vi "Login Dialog.vi"() -> (0 "管理员":bool, 2 "Success?":bool)   [LabVIEW 2015]
uses:
  <vilib>/Utility/miscctls.llb/LVPointTypeDef.ctl
  Global.vi
panel:
  in  "注册":bool
  in  "登录":bool
  in  "注销":bool
  in  "Password":string caption="密   码:"
  in  "UserName":string caption="用户名:"
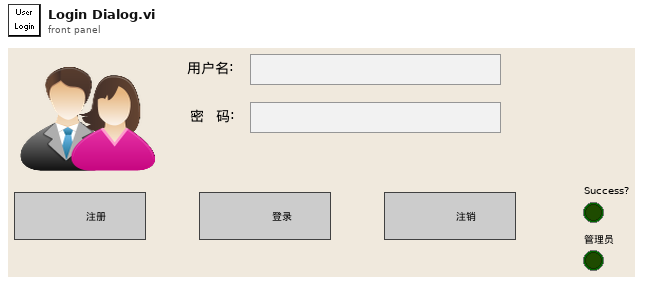
[diagram p1: front panel]
types:
  T1 = typedef "LVPointTypeDef.ctl" = cluster{"Horizontal":i16, "Vertical":i16}
  T2 = enum8{"Enabled", "Disabled", "Disabled and Grayed Out"}
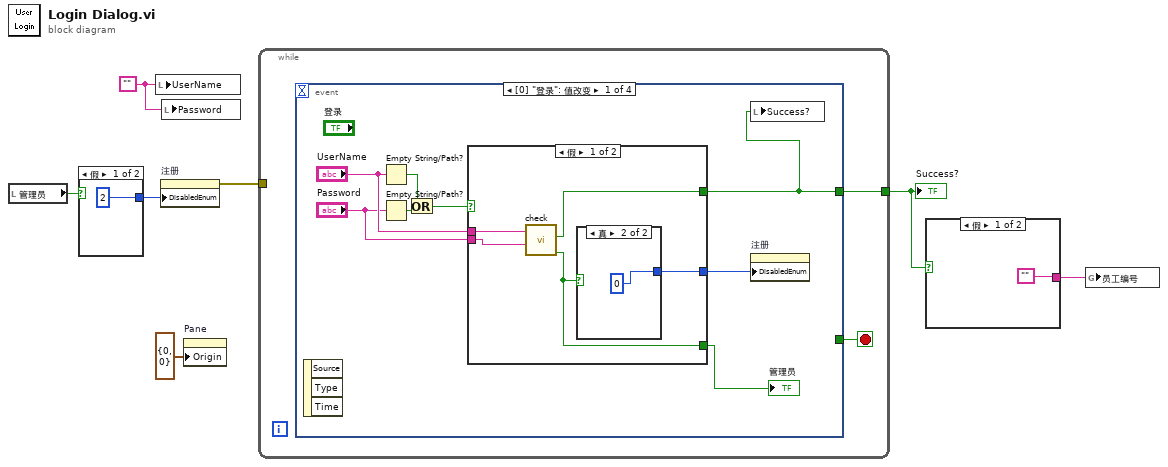
[diagram p0: block diagram]
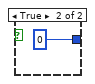
[diagram p2: hidden frame]
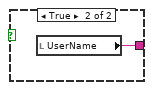
[diagram p3: hidden frame]
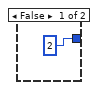
[diagram p4: hidden frame]
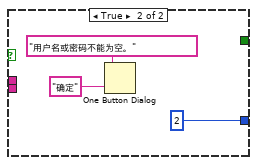
[diagram p5: hidden frame]
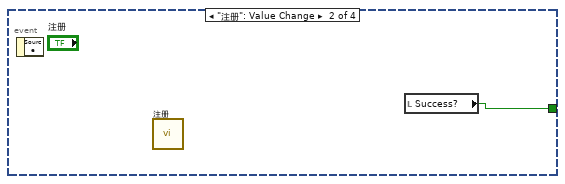
[diagram p6: hidden frame]
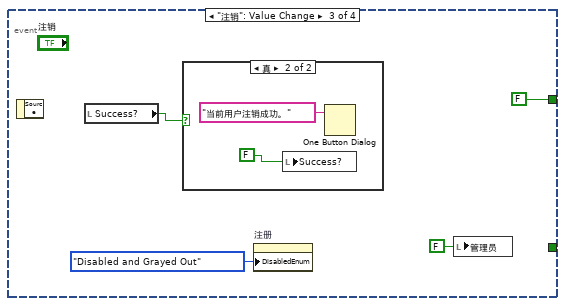
[diagram p7: hidden frame]
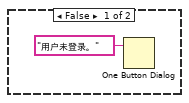
[diagram p8: hidden frame]
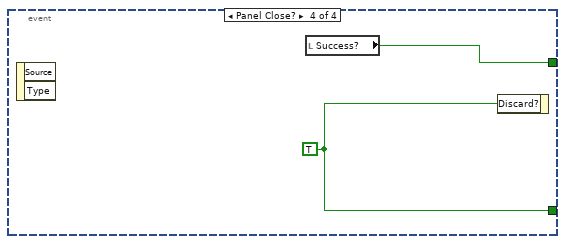
[diagram p9: hidden frame]
diagram:
  w6 = ""
  n1 = local read "管理员"() -> (w3:bool)
  n2 = case shown="假" w3 {
    tunnel: [2 0] -> w2
    frame False {
    }
    frame True {
    }
  }
  n3 = local write "UserName"(w6) -> ()
  n4 = property on="注册" class="Bool"("DisabledEnum"=w2) -> (error out=w1:errorcluster)  [unwired: 2 in, 1 out]
  n5 = local write "Password"(w6) -> ()
  n6 = property on="Pane" class="Pane"("Origin"=T1 {"Horizontal"=0, "Vertical"=0}) -> ()  [unwired: 2 in, 2 out]
  n7 = while {
    tunnel: [w10] -> w5
    tunnel: w1 -> [_]
    stop <- w11 stop-if-true
    n8 = event shown="[0] \"登录\": 值改变" {
      selector: _ -> [_ _ _ _]
      dyn-events: _ -> [_ _ _ _]
      timeout: _ -> [_ _ _ _]
      tunnel: [_ _ _ w39] -> w11
      tunnel: [w14 w30 FALSE ("Success?") w38] -> w10
      event "登录": Value Change {
        n9 = event-data() -> ()  [unwired: 1 in, 3 out]
        n10 = Empty String/Path?(string/path="UserName") -> (empty?=w18:bool)
        n11 = Empty String/Path?(string/path="Password") -> (empty?=w19:bool)
        n12 = Or(x=w18, y=w19) -> (x .or. y?=w17:bool)
        n13 = case shown="假" w17 {
          tunnel: "UserName" -> [w24 _]
          tunnel: "Password" -> [w23 _]
          tunnel: [w22 _] -> w14
          tunnel: [w21 2] -> w13
          tunnel: [w20 _] -> w12
          frame False {
            n14 = call "check.vi"("Password"=w23, "UserName"=w24) -> ("管理员"=w20:bool, "Success?"=w22:bool)  [unwired: 8 in]
            n15 = case shown="真" w20 {
              tunnel: [2 0] -> w21
              frame False {
              }
              frame True {
              }
            }
          }
          frame True {
            n16 = One Button Dialog(message="用户名或密码不能为空。", button name ("OK")="确定") -> ()  [unwired: 1 out]
          }
        }
        "管理员" <- w12
        n17 = local write "Success?"(w14) -> ()
        n18 = property on="注册" class="Bool"("DisabledEnum"=w13) -> ()  [unwired: 2 in, 2 out]
      }
      event "注册": Value Change {
        n19 = event-data() -> ()  [unwired: 1 in, 1 out]
        n20 = call "注册.vi"() -> ()  [unwired: 12 in]
        n21 = local read "Success?"() -> (w30:bool)
      }
      event "注销": Value Change {
        n22 = event-data() -> ()  [unwired: 1 in, 1 out]
        n23 = local read "Success?"() -> (w33:bool)
        n24 = case shown="真" w33 {
          frame False {
            n25 = One Button Dialog(message="用户未登录。" ("消息")) -> ()  [unwired: 1 in, 1 out]
          }
          frame True {
            n26 = local write "Success?"(FALSE ("Success?")) -> ()
            n27 = One Button Dialog(message="当前用户注销成功。" ("消息")) -> ()  [unwired: 1 in, 1 out]
          }
        }
        n28 = property on="注册" class="Bool"("DisabledEnum"=T2."Disabled and Grayed Out" ("禁用")) -> ()  [unwired: 2 in, 2 out]
        n29 = local write "管理员"(FALSE ("管理员")) -> ()
      }
      event Panel Close? {
        w39 = TRUE
        n30 = event-data() -> ()  [unwired: 1 in, 2 out]
        n31 = local read "Success?"() -> (w38:bool)
        n32 = event-data("Discard?"=w39) -> ()  [unwired: 1 in, 1 out]
      }
    }
  }
  "Success?" <- w5
  n33 = case shown="假" w5 {
    tunnel: ["" w41] -> w4
    frame False {
    }
    frame True {
      n34 = local read "UserName"() -> (w41:string)
    }
  }
  n35 = global write "Global.vi" "员工编号"(w4) -> ()
